vi "Page_Source_Add.vi"(4 "ctlReferences":T2, 6 "sourceInclusion":T1, 7 "items to add in":string[](array[string]), 8 "error in (no error)":errorcluster, 9 "send to main dest?":bool, 10 "Project Refnum":refnum<vi>, 11 "AB_Source_Container in":refnum<class "AB_Source_Container.lvclass">) -> (0 "error out":errorcluster, 2 "changed":bool, 3 "AB_Source_Container out":refnum<class "AB_Source_Container.lvclass">, 5 "items to add out":string[](array[string]))   [LabVIEW 2020, in "AB_Source_Container.lvclass"]
uses:
  <vilib>/AppBuilder/AB_Classes/Source/Container/AB_Source_Container.lvclass
  e:/builds/penguin/labview/branches/2020/dev/dist/vi.lib/AppBuilder/AB_Classes/Source/AB_Source.lvclass
  <resource>/Framework/Providers/Builds/AppBuilder/AB_UI_Page_Source_Files_References.ctl
  <vilib>/AppBuilder/AB_Source_Inclusion.ctl
  <vilib>/AppBuilder/AB_Classes/Source/AB_Source.lvclass
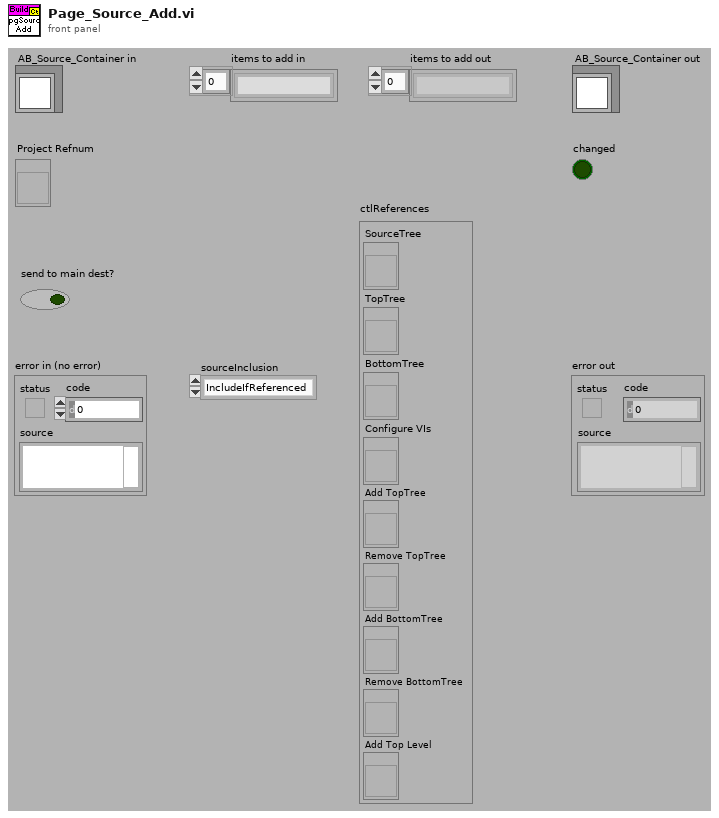
[diagram p1: front panel]
types:
  T1 = typedef "AB_Source_Inclusion.ctl" = enum16{"IncludeIfReferenced", "Include", "Exclude", "TopLevel"}
  T2 = typedef "AB_UI_Page_Source_Files_References.ctl" = cluster{"SourceTree":refnum<vi>, "TopTree":refnum<vi>, "BottomTree":refnum<vi>, "Configure VIs":refnum<vi>, "Add TopTree":refnum<vi>, "Remove TopTree":refnum<vi>, "Add BottomTree":refnum<vi>, "Remove BottomTree":refnum<vi>, "Add Top Level":refnum<vi>}
  T3 = typedef "AB_Source_Container.ctl" = cluster{"applyInclusion":bool, "applyDestination":bool, "applyProperties":bool, "applyPassword":bool, "applyPrefix":bool, "applySaveSetttings":bool, "dependentDestinationIndex":i32}
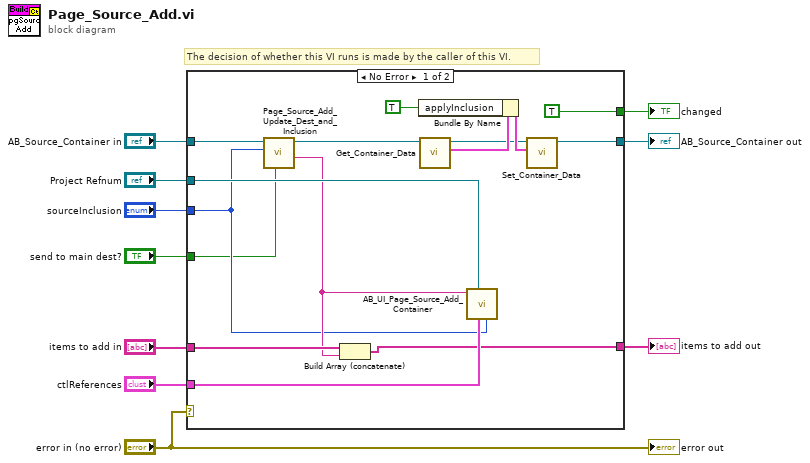
[diagram p0: block diagram]
diagram:
  # "The decision of whether this VI runs is made by the caller of this VI."
  n1 = case shown="No Error" "error in (no error)" {
    tunnel: "AB_Source_Container in" -> [w25 w26]
    tunnel: [w24 w26] -> w9
    tunnel: [TRUE _] -> w8
    tunnel: "Project Refnum" -> [w22 _]
    tunnel: "ctlReferences" -> [w21 _]
    tunnel: "send to main dest?" -> [w11 _]
    tunnel: "items to add in" -> [w20 _]
    tunnel: [w19 _] -> w2
    tunnel: "sourceInclusion" -> [w12 _]
    frame No Error {
      n2 = call <vilib>:"Page_Source_Add_Update_Dest_and_Inclusion.vi"("send to main destination?"=w11, "Inclusion"=w12, "AB_Source_VI in"=w25) -> ("itemID"=w13:string, "AB_Source_VI out"=w14:refnum<class "AB_Source_Container.lvclass">)  [unwired: 6 in, 1 out]
      n3 = Build Array (concatenate)(w20, w13) -> (w19:string[])
      n4 = call <vilib>:"Get_Container_Data.vi"("Class in"=w14) -> ("data"=w18:T3, "Class out"=w15:refnum<class "AB_Source_Container.lvclass">)  [unwired: 8 in, 1 out]
      n5 = Bundle By Name(cluster=w18, "applyInclusion"=TRUE) -> (w17:T3)
      n6 = call <resource>:"AB_UI_Page_Source_Add_Container.vi"("sourceInclusion"=w12, "ctlReferences"=w21, "Project Refnum"=w22, "itemID"=w13) -> ()  [unwired: 7 in, 1 out]
      n7 = call <vilib>:"Set_Container_Data.vi"("data"=w17, "Class in"=w15) -> ("Class out"=w24:refnum<class "AB_Source_Container.lvclass">)  [unwired: 8 in, 1 out]
    }
    frame Error {
    }
  }
  "changed" <- w8
  "AB_Source_Container out" <- w9
  "items to add out" <- w2
  "error out" <- "error in (no error)"
